vi "DriveForDistance-C.vi"(11 "Params":string[][](array[string])) -> ()   [LabVIEW 2017]
uses:
  Framework/Robot Global Data.vi
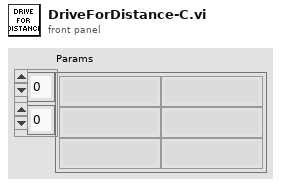
[diagram p1: front panel]
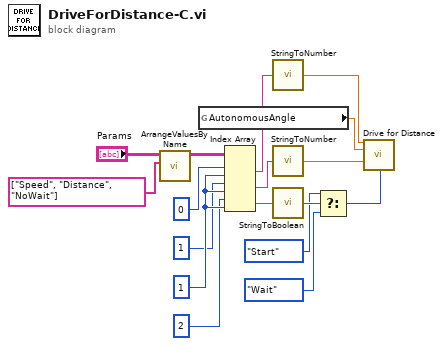
[diagram p0: block diagram]
diagram:
  w6 = 1
  n1 = call "ArrangeValuesByName.vi"("Names"=string[] ["Speed", "Distance", "NoWait"], "Names/Values in"="Params") -> ("Names/Values Out"=w8:string[][])  [unwired: 9 in]
  n2 = global read "Robot Global Data.vi" "AutonomousAngle"() -> (w15:dbl)
  n3 = Index Array(array=w8, index (row) #1=0, index (col) #1=w6, index (row) #2=1, index (col) #2=w6, index (row) #3=2, index (col) #3=w6) -> (element #1=w3:string, element #2=w2:string, element #3=w1:string)
  n4 = call "StringToNumber.vi"("String"=w3) -> ("Output"=w17:dbl)
  n5 = call "StringToNumber.vi"("String"=w2) -> ("Output"=w16:dbl)
  n6 = call "StringToBoolean.vi"("String"=w1) -> ("Output"=w14:bool)
  n7 = Select(t=enum16{"Start", "Wait"}."Start", s=w14, f=enum16{"Start", "Wait"}."Wait" ("Synchronication")) -> (s? t:f=w11:enum16{"Start", "Wait"})
  n8 = call "Drive for Distance.vi"("Speed"=w17, "StartAngle"=w15, "Distance (inch)"=w16, "Synchronication"=w11) -> ()  [unwired: 11 in, 1 out]
